vi "Write Context.vi"(10 "Context":string, 11 "Network Stream in":refnum<class "Network Stream.lvclass">) -> (3 "Network Stream out":refnum<class "Network Stream.lvclass">)   [LabVIEW 2020, in "Network Stream.lvclass"]
doc: "Use this VI to specify the IP address for this endpoint of the network stream."
uses:
  Network Stream.lvclass
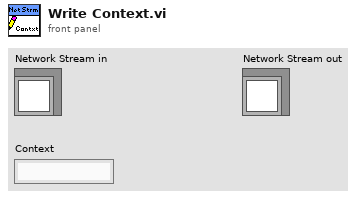
[diagram p1: front panel]
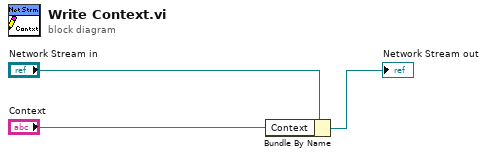
[diagram p0: block diagram]
diagram:
  n1 = Bundle By Name(cluster="Network Stream in", "Context"="Context") -> (→"Network Stream out":refnum<class "Network Stream.lvclass">)
